vi "Check Boundary.vi"(9 "Gate Condition":bool[](array[boolean]), 10 "Collision Box":T1={"left"=375, "top"=375, "right"=425, "bottom"=425}, 11 "Bounding Case":T2) -> (1 "Move?":bool)   [LabVIEW 2025]
uses:
  Bounding Case.ctl
  Collision Box.ctl
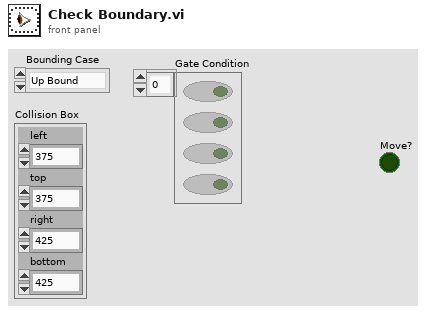
[diagram p1: front panel]
types:
  T1 = typedef "Collision Box.ctl" = cluster{"left":i16, "top":i16, "right":i16, "bottom":i16}
  T2 = typedef "Bounding Case.ctl" = enum16{"Up Bound", "Down Bound", "Left Bound", "Right Bound"}
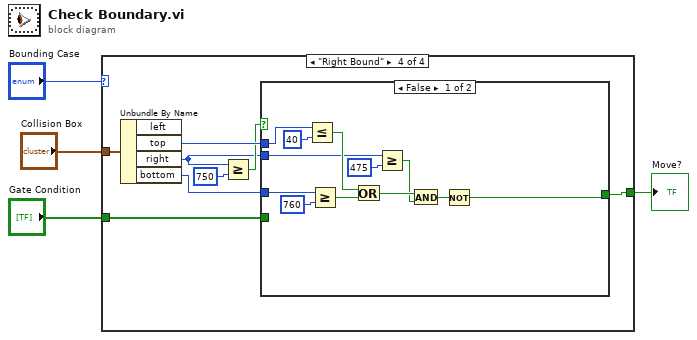
[diagram p0: block diagram]
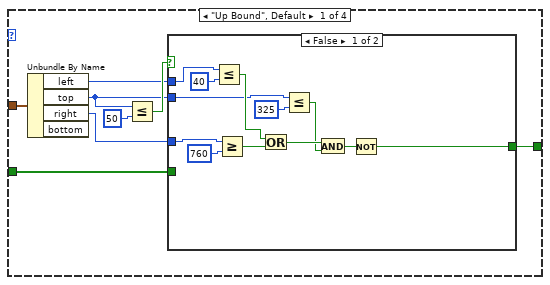
[diagram p2: hidden frame]
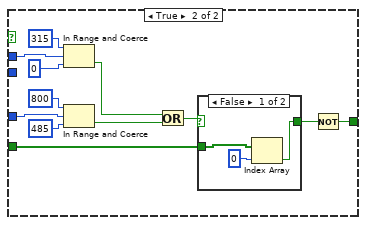
[diagram p3: hidden frame]
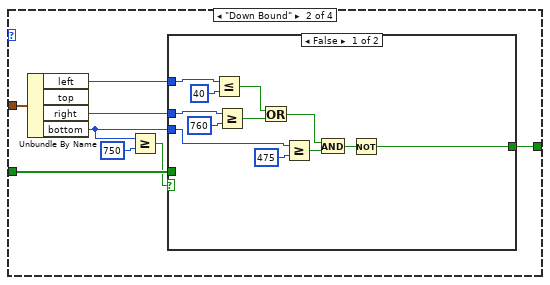
[diagram p5: hidden frame]
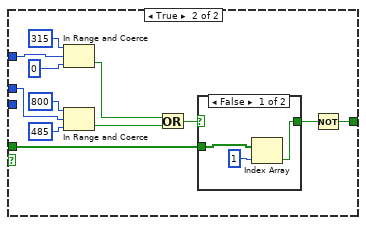
[diagram p6: hidden frame]
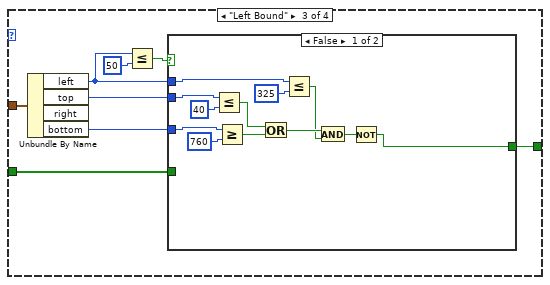
[diagram p8: hidden frame]
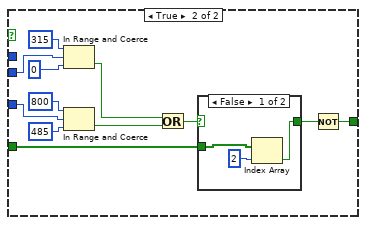
[diagram p9: hidden frame]
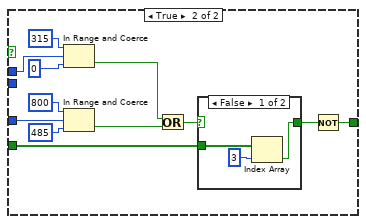
[diagram p11: hidden frame]
diagram:
  n1 = case shown="\"Right Bound\"" "Bounding Case" {
    tunnel: "Collision Box" -> [w12 w45 w78 w114]
    tunnel: "Gate Condition" -> [w6 w46 w84 w118]
    tunnel: [w9 w44 w83 w117] -> w1
    frame "Up Bound", Default {
      n2 = Unbundle By Name(w12) -> ("left"=w8:i16, "top"=w5:i16, "right"=w7:i16)  [unwired: 1 out]
      n3 = Less Or Equal?(x=w5, y=i16 50) -> (x <= y?=w10:bool)
      n4 = case shown="False" w10 {
        tunnel: [w13 w25] -> w9
        tunnel: w8 -> [w24 w36]
        tunnel: w7 -> [w21 w33]
        tunnel: w6 -> [_ w27]
        tunnel: w5 -> [w17 _]
        frame False {
          n5 = Less Or Equal?(x=w24, y=i16 40) -> (x <= y?=w22:bool)
          n6 = Greater Or Equal?(x=w21, y=i16 760) -> (x >= y?=w19:bool)
          n7 = Or(x=w22, y=w19) -> (x .or. y?=w18:bool)
          n8 = Less Or Equal?(x=w17, y=i16 325) -> (x <= y?=w15:bool)
          n9 = And(x=w18, y=w15) -> (x .and. y?=w14:bool)
          n10 = Not(x=w14) -> (.not. x?=w13:bool)
        }
        frame True {
          n11 = In Range and Coerce(upper limit=i16 315, x=w36, lower limit=i16 0) -> (In Range?=w29:bool)  [unwired: 1 out]
          n12 = In Range and Coerce(upper limit=i16 800, x=w33, lower limit=i16 485) -> (In Range?=w30:bool)  [unwired: 1 out]
          n13 = Or(x=w29, y=w30) -> (x .or. y?=w28:bool)
          n14 = case shown="False" w28 {
            selector: w28 -> [_ w40]
            tunnel: [w37 w40] -> w26
            tunnel: w27 -> [w39 _]
            frame False {
              n15 = Index Array(array=w39, index=0) -> (element=w37:bool)
            }
            frame True {
            }
          }
          n16 = Not(x=w26) -> (.not. x?=w25:bool)
        }
      }
    }
    frame "Down Bound" {
      n17 = Unbundle By Name(w45) -> ("left"=w48:i16, "right"=w47:i16, "bottom"=w41:i16)  [unwired: 1 out]
      n18 = Greater Or Equal?(x=w41, y=i16 750) -> (x >= y?=w43:bool)
      n19 = case shown="False" w43 {
        tunnel: [w54 w61] -> w44
        tunnel: w48 -> [w53 w72]
        tunnel: w47 -> [w52 w69]
        tunnel: w46 -> [_ w63]
        tunnel: w41 -> [w50 _]
        frame False {
          n20 = Less Or Equal?(x=w53, y=i16 40) -> (x <= y?=w59:bool)
          n21 = Greater Or Equal?(x=w52, y=i16 760) -> (x >= y?=w57:bool)
          n22 = Or(x=w59, y=w57) -> (x .or. y?=w56:bool)
          n23 = Greater Or Equal?(x=w50, y=i16 475) -> (x >= y?=w51:bool)
          n24 = And(x=w56, y=w51) -> (x .and. y?=w55:bool)
          n25 = Not(x=w55) -> (.not. x?=w54:bool)
        }
        frame True {
          n26 = In Range and Coerce(upper limit=i16 315, x=w72, lower limit=i16 0) -> (In Range?=w65:bool)  [unwired: 1 out]
          n27 = In Range and Coerce(upper limit=i16 800, x=w69, lower limit=i16 485) -> (In Range?=w66:bool)  [unwired: 1 out]
          n28 = Or(x=w65, y=w66) -> (x .or. y?=w64:bool)
          n29 = case shown="False" w64 {
            selector: w64 -> [_ w76]
            tunnel: [w73 w76] -> w62
            tunnel: w63 -> [w75 _]
            frame False {
              n30 = Index Array(array=w75, index=1) -> (element=w73:bool)
            }
            frame True {
            }
          }
          n31 = Not(x=w62) -> (.not. x?=w61:bool)
        }
      }
    }
    frame "Left Bound" {
      n32 = Unbundle By Name(w78) -> ("left"=w77:i16, "top"=w82:i16, "bottom"=w81:i16)  [unwired: 1 out]
      n33 = Less Or Equal?(x=w77, y=i16 50) -> (x <= y?=w80:bool)
      n34 = case shown="False" w80 {
        tunnel: [w90 w97] -> w83
        tunnel: w82 -> [w89 w108]
        tunnel: w81 -> [w88 w105]
        tunnel: w84 -> [_ w99]
        tunnel: w77 -> [w85 _]
        frame False {
          n35 = Less Or Equal?(x=w89, y=i16 40) -> (x <= y?=w95:bool)
          n36 = Greater Or Equal?(x=w88, y=i16 760) -> (x >= y?=w93:bool)
          n37 = Or(x=w95, y=w93) -> (x .or. y?=w92:bool)
          n38 = Less Or Equal?(x=w85, y=i16 325) -> (x <= y?=w87:bool)
          n39 = And(x=w92, y=w87) -> (x .and. y?=w91:bool)
          n40 = Not(x=w91) -> (.not. x?=w90:bool)
        }
        frame True {
          n41 = In Range and Coerce(upper limit=i16 315, x=w108, lower limit=i16 0) -> (In Range?=w101:bool)  [unwired: 1 out]
          n42 = In Range and Coerce(upper limit=i16 800, x=w105, lower limit=i16 485) -> (In Range?=w102:bool)  [unwired: 1 out]
          n43 = Or(x=w101, y=w102) -> (x .or. y?=w100:bool)
          n44 = case shown="False" w100 {
            selector: w100 -> [_ w112]
            tunnel: [w109 w112] -> w98
            tunnel: w99 -> [w111 _]
            frame False {
              n45 = Index Array(array=w111, index=2) -> (element=w109:bool)
            }
            frame True {
            }
          }
          n46 = Not(x=w98) -> (.not. x?=w97:bool)
        }
      }
    }
    frame "Right Bound" {
      n47 = Unbundle By Name(w114) -> ("top"=w120:i16, "right"=w113:i16, "bottom"=w119:i16)  [unwired: 1 out]
      n48 = Greater Or Equal?(x=w113, y=i16 750) -> (x >= y?=w115:bool)
      n49 = case shown="False" w115 {
        tunnel: [w124 w133] -> w117
        tunnel: w120 -> [w123 w144]
        tunnel: w119 -> [w122 w141]
        tunnel: w118 -> [_ w135]
        tunnel: w113 -> [w121 _]
        frame False {
          n50 = Less Or Equal?(x=w123, y=i16 40) -> (x <= y?=w131:bool)
          n51 = Greater Or Equal?(x=w122, y=i16 760) -> (x >= y?=w129:bool)
          n52 = Or(x=w131, y=w129) -> (x .or. y?=w128:bool)
          n53 = Greater Or Equal?(x=w121, y=i16 475) -> (x >= y?=w126:bool)
          n54 = And(x=w128, y=w126) -> (x .and. y?=w127:bool)
          n55 = Not(x=w127) -> (.not. x?=w124:bool)
        }
        frame True {
          n56 = In Range and Coerce(upper limit=i16 315, x=w144, lower limit=i16 0) -> (In Range?=w137:bool)  [unwired: 1 out]
          n57 = In Range and Coerce(upper limit=i16 800, x=w141, lower limit=i16 485) -> (In Range?=w138:bool)  [unwired: 1 out]
          n58 = Or(x=w137, y=w138) -> (x .or. y?=w136:bool)
          n59 = case shown="False" w136 {
            selector: w136 -> [_ w148]
            tunnel: [w145 w148] -> w134
            tunnel: w135 -> [w147 _]
            frame False {
              n60 = Index Array(array=w147, index=3) -> (element=w145:bool)
            }
            frame True {
            }
          }
          n61 = Not(x=w134) -> (.not. x?=w133:bool)
        }
      }
    }
  }
  "Move?" <- w1
